vi "Wait syringe pump.vi"(8 "error in (no error)":errorcluster, 10 "Delayed time (s)":dbl, 11 "Time Target (s)":dbl=1.0) -> (0 "error out":errorcluster)   [LabVIEW 2017]
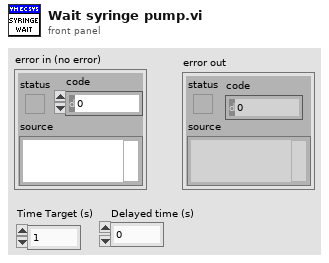
[diagram p1: front panel]
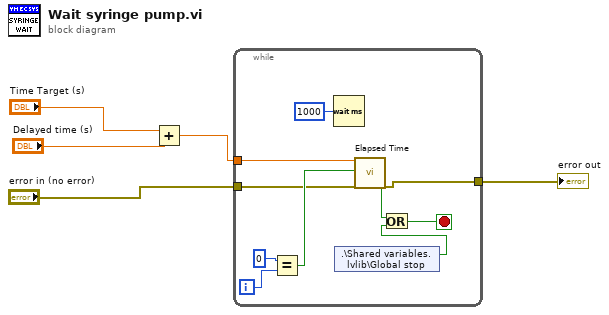
[diagram p0: block diagram]
diagram:
  n1 = Add(x="Time Target (s)", y="Delayed time (s)") -> (x+y=w2:dbl)
  n2 = while {
    tunnel: w2 -> [w9]
    tunnel: "error in (no error)" -> [w8]
    tunnel: [w7] -> w1
    i -> [w15]
    stop <- w12 stop-if-true
    n3 = Equal?(x=0, y=w15) -> (x = y?=w13:bool)
    n4 = Wait (ms)(milliseconds to wait=u32 1000) -> ()  [unwired: 1 out]
    n5 = shared-variable ".\\Shared variables.lvlib\\Global stop"() -> (w10:bool)  [unwired: 1 in, 1 out]
    n6 = call "Elapsed Time"("Time Target (s)"=w9, "Reset"=w13, "error in (no error)"=w8) -> ("Time has Elapsed"=w11:bool, "error out"=w7:errorcluster)  [unwired: 9 in, 6 out]
    n7 = Or(x=w11, y=w10) -> (x .or. y?=w12:bool)
  }
  "error out" <- w1
